vi "Tosca-Remap TTL Outputs.vi"(0 "Tosca":refnum<class "Parameters.lvclass">, 7 "FSM.Graph In":refnum<class "FSM.Graph.lvclass">, 11 "error in (no error)":errorcluster) -> (4 "Tosca out":refnum<class "Parameters.lvclass">, 8 "FSM.Graph Out":refnum<class "FSM.Graph.lvclass">, 10 "remapped":bool, 15 "error IO":errorcluster)   [LabVIEW 2020]
uses:
  Classes/Parameters/Parameters.lvclass
  FSM Graph VIs/LV Source/Classes/FSM.Graph/FSM.Graph.lvclass
  TTL VIs/Device Classes/Base Class/TTLControlledDevice.lvclass
  TTL VIs/Device Classes/Base Class/TTLControlledDevice.lvclass/TTLControlledDevice.ctl
  TTL VIs/Device Classes/Base Class/Read Name.vi
  Tosca-Globals.vi
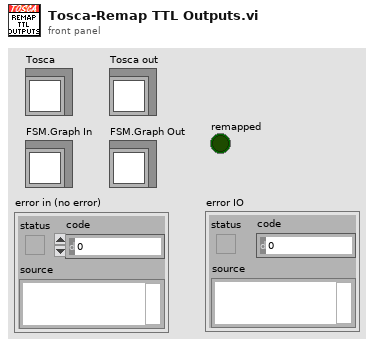
[diagram p1: front panel]
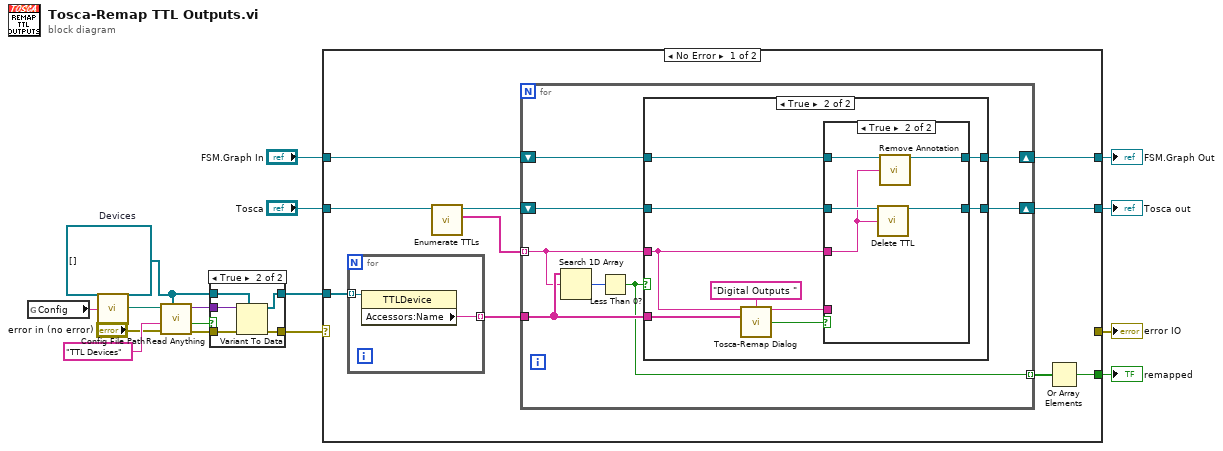
[diagram p0: block diagram]
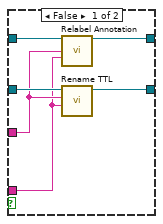
[diagram p4: hidden frame]
diagram:
  w8 = refnum<class "TTLControlledDevice.lvclass">[] []  # Devices
  n1 = global read "Tosca-Globals.vi" "Config"() -> (w15:string)
  n2 = call "Config File Path.vi"("AppName"=w15) -> ("Default config file name"=w6:path)
  n3 = call "Read Anything.vi"("Type of Anything"=w8, "Error In"="error in (no error)", "Section Name (Name of \"Type of Anything\")"="TTL Devices" ("Section Name (Name of \"Type of Anything\")"), "Path (dialog)"=w6) -> ("Error Out"=w11:errorcluster, "Found?"=w9:bool, "Anything"=w10:variant)  [unwired: 5 in]
  n4 = case shown="True" w9 {
    tunnel: w11 -> [w17 w23]
    tunnel: w10 -> [_ w22]
    tunnel: w8 -> [w18 w21]
    tunnel: [w18 w20] -> w4
    tunnel: [w17 w19] -> w5
    frame False {
    }
    frame True {
      n5 = Variant To Data(error in=w23, type=w21, Variant=w22) -> (data=w20:refnum<class "TTLControlledDevice.lvclass">[], error out=w19:errorcluster)
    }
  }
  n6 = case shown="No Error" w5 {
    selector: w5 -> [_ w68]
    tunnel: [_ w68] -> w16
    tunnel: "Tosca" -> [w33 w67]
    tunnel: [w30 w67] -> w13
    tunnel: w4 -> [w29 _]
    tunnel: [w26 _] -> w3
    tunnel: "FSM.Graph In" -> [w25 w66]
    tunnel: [w24 w66] -> w1
    frame No Error {
      n7 = for {
        tunnel: w29 -> [w35] mode=indexing
        tunnel: [w34] -> w28 mode=indexing
        n8 = property class="TTLDevice"(reference=w35) -> ("Accessors:Name"=w34:string)  [unwired: 1 in, 2 out]
      }
      n9 = call "Enumerate TTLs.vi"("Tosca in"=w33) -> ("Endpoints"=w32:string[], "Tosca out"=w31:refnum<class "Parameters.lvclass">)  [unwired: 8 in, 1 out]
      n10 = for {
        tunnel: w28 -> [w43]
        tunnel: w32 -> [w41] mode=indexing
        shift-right: [w39] -> w30
        shift-left: w31 -> [w40]
        tunnel: [w38] -> w27 mode=indexing
        shift-right: [w36] -> w24
        shift-left: w25 -> [w37]
        n11 = Search 1D Array(1D array=w43, element=w41) -> (index of element=w42:i32)  [unwired: 1 in]
        n12 = Less Than 0?(x=w42) -> (x < 0?=w38:bool)
        n13 = case shown="True" w38 {
          tunnel: w43 -> [_ w53]
          tunnel: w41 -> [_ w49]
          tunnel: w40 -> [w45 w52]
          tunnel: [w45 w48] -> w39
          tunnel: w37 -> [w44 w47]
          tunnel: [w44 w46] -> w36
          frame False {
          }
          frame True {
            n14 = call "Tosca-Remap Dialog.vi"("Old Name In"=w49, "Type"="Digital Outputs ", "New Names"=w53) -> ("Old Name Out"=w50:string, "Deleted?"=w51:bool)  [unwired: 10 in, 1 out]
            n15 = case shown="True" w51 {
              tunnel: w52 -> [w60 w65]
              tunnel: w50 -> [w55 _]
              tunnel: w49 -> [w56 w61]
              tunnel: [w59 w64] -> w48
              tunnel: w47 -> [w58 w63]
              tunnel: [w57 w62] -> w46
              frame False {
                n16 = call "Relabel Annotation.vi"("FSM.Graph In"=w58, "Old Name"=w56, "New Name"=w55) -> ("FSM.Graph Out"=w57:refnum<class "FSM.Graph.lvclass">)  [unwired: 12 in]
                n17 = call "Rename TTL.vi"("New name"=w55, "Old name"=w56, "Tosca in"=w60) -> ("Tosca out"=w59:refnum<class "Parameters.lvclass">)  [unwired: 7 in, 1 out]
              }
              frame True {
                n18 = call "Delete TTL.vi"("Tosca in"=w65, "Name"=w61) -> ("Tosca out"=w64:refnum<class "Parameters.lvclass">)  [unwired: 12 in, 1 out]
                n19 = call "Remove Annotation.vi"("FSM.Graph In"=w63, "Name"=w61) -> ("FSM.Graph Out"=w62:refnum<class "FSM.Graph.lvclass">)  [unwired: 13 in]
              }
            }
          }
        }
      }
      n20 = Or Array Elements(Boolean array=w27) -> (logical OR=w26:bool)
    }
    frame Error {
    }
  }
  "error IO" <- w16
  "Tosca out" <- w13
  "remapped" <- w3
  "FSM.Graph Out" <- w1
